vi "draw_3d_scene.vi"(4 "park plane z (px)":dbl=100.0, 5 "cells":dbl[][](array[numeric]), 6 "manip 4":dbl[][](array[numeric]), 7 "manip 1":dbl[][](array[numeric]), 8 "error in":errorcluster, 9 "manip 3":dbl[][](array[numeric]), 10 "manip 2":dbl[][](array[numeric]), 11 "3d graph":refnum<k7>) -> (0 "error out":errorcluster, 3 "currentState out":T1(array[cluster]))   [LabVIEW 2015]
uses:
  <vilib>/Platform/NI_3dgraph.lvlib
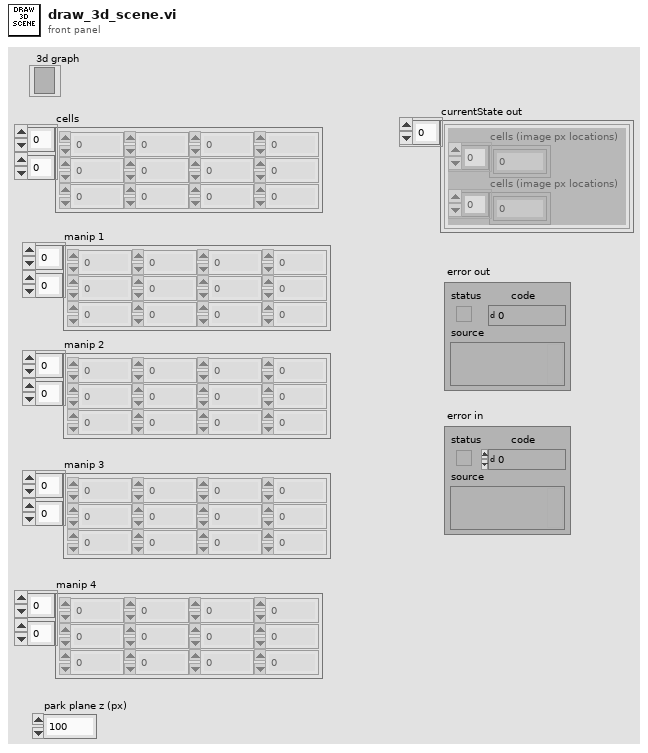
[diagram p1: front panel]
types:
  T1 = cluster{"cells (image px locations)":dbl[], "cells (image px locations)":dbl[]}[]
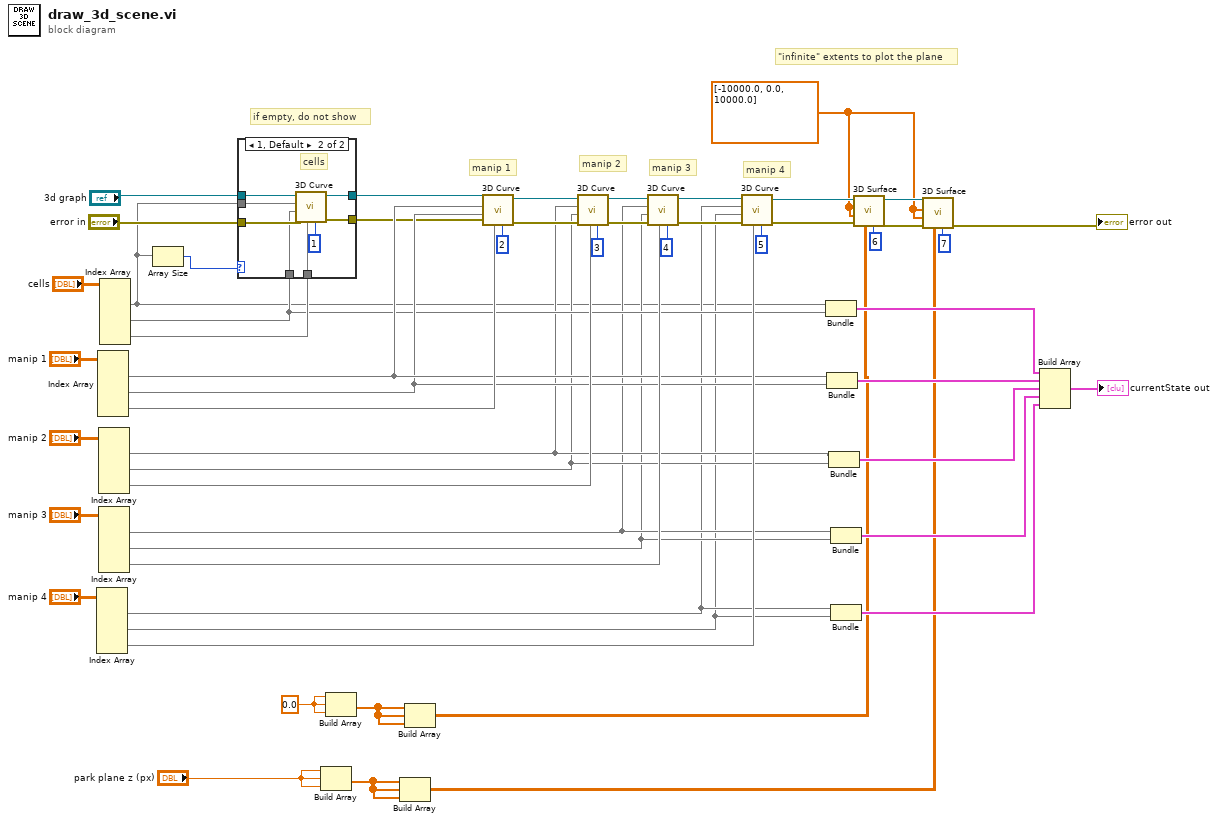
[diagram p0: block diagram]
diagram:
  w13 = 0.0 ("element")
  w6 = dbl[] [-10000.0, 0.0, 10000.0] ("x vector")
  # "if empty, do not show"
  # "\"infinite\" extents to plot the plane"
  # "manip 4"
  # "manip 3"
  # "manip 2"
  # "manip 1"
  n1 = Index Array(array="manip 4") -> (element #1=w21:dbl[], element #2=w20:dbl[], element #3=w41:dbl[])  [unwired: 6 in]
  n2 = Index Array(array="manip 1") -> (element #1=w36:dbl[], element #2=w35:dbl[], element #3=w47:dbl[])  [unwired: 6 in]
  n3 = Index Array(array="manip 2") -> (element #1=w26:dbl[], element #2=w25:dbl[], element #3=w43:dbl[])  [unwired: 6 in]
  n4 = Index Array(array="manip 3") -> (element #1=w23:dbl[], element #2=w22:dbl[], element #3=w42:dbl[])  [unwired: 6 in]
  n5 = Index Array(array="cells") -> (element #1=w1:dbl[], element #2=w28:dbl[], element #3=w29:dbl[])  [unwired: 6 in]
  n6 = Array Size(array=w1) -> (size(s)=w3:i32)
  n7 = case shown="1, Default" w3 {
    tunnel: "3d graph" -> [w57 w65]
    tunnel: "error in" -> [w56 w64]
    tunnel: [w56 w63] -> w31
    tunnel: [w57 w61] -> w30
    tunnel: w29 -> [_ w60]
    tunnel: w1 -> [_ w59]
    tunnel: w28 -> [_ w58]
    frame 0 {
    }
    frame 1, Default {
      # "cells"
      n8 = call <vilib>:"3D Curve.vi"("plot number (1)"=1, "z vector"=w60, "error in (no error)"=w64, "y vector"=w58, "x vector"=w59, "3D graph"=w65) -> ("error out"=w63:errorcluster, "3D graph out"=w61:refnum<k7>)  [unwired: 4 in]
    }
  }
  n9 = Build Array("park plane z (px)", "park plane z (px)", "park plane z (px)") -> (w9:dbl[])
  n10 = Build Array(w13, w13, w13) -> (w15:dbl[])
  n11 = Build Array(w9, w9, w9) -> (w7:dbl[][])
  n12 = Build Array(w15, w15, w15) -> (w14:dbl[][])
  n13 = call <vilib>:"3D Curve.vi"("plot number (1)"=2, "z vector"=w47, "error in (no error)"=w31, "y vector"=w35, "x vector"=w36, "3D graph"=w30) -> ("error out"=w49:errorcluster, "3D graph out"=w55:refnum<k7>)  [unwired: 4 in]
  n14 = call <vilib>:"3D Curve.vi"("plot number (1)"=3, "z vector"=w43, "error in (no error)"=w49, "y vector"=w25, "x vector"=w26, "3D graph"=w55) -> ("error out"=w39:errorcluster, "3D graph out"=w50:refnum<k7>)  [unwired: 4 in]
  n15 = call <vilib>:"3D Curve.vi"("plot number (1)"=4, "z vector"=w42, "error in (no error)"=w39, "y vector"=w22, "x vector"=w23, "3D graph"=w50) -> ("error out"=w38:errorcluster, "3D graph out"=w40:refnum<k7>)  [unwired: 4 in]
  n16 = call <vilib>:"3D Curve.vi"("plot number (1)"=5, "z vector"=w41, "error in (no error)"=w38, "y vector"=w20, "x vector"=w21, "3D graph"=w40) -> ("error out"=w16:errorcluster, "3D graph out"=w17:refnum<k7>)  [unwired: 4 in]
  n17 = Bundle("cells"=w1, "cells"=w28) -> (w27:cluster{"cells":dbl[], "cells":dbl[]})  [unwired: 1 in]
  n18 = Bundle("manip 1"=w36, "manip 1"=w35) -> (w34:cluster{"manip 1":dbl[], "manip 1":dbl[]})  [unwired: 1 in]
  n19 = Bundle("manip 2"=w26, "manip 2"=w25) -> (w24:cluster{"manip 2":dbl[], "manip 2":dbl[]})  [unwired: 1 in]
  n20 = Bundle("manip 3"=w23, "manip 3"=w22) -> (w19:cluster{"manip 3":dbl[], "manip 3":dbl[]})  [unwired: 1 in]
  n21 = Bundle("manip 4"=w21, "manip 4"=w20) -> (w18:cluster{"manip 4":dbl[], "manip 4":dbl[]})  [unwired: 1 in]
  n22 = call <vilib>:"3D Surface.vi"("plot number (1)"=6, "z matrix"=w14, "error in (no error)"=w16, "y vector"=w6, "x vector"=w6, "3D graph"=w17) -> ("error out"=w12:errorcluster, "3D graph out"=w10:refnum<k7>)  [unwired: 4 in]
  n23 = call <vilib>:"3D Surface.vi"("plot number (1)"=7, "z matrix"=w7, "error in (no error)"=w12, "y vector"=w6, "x vector"=w6, "3D graph"=w10) -> ("error out"=→"error out":errorcluster)  [unwired: 4 in, 1 out]
  n24 = Build Array(w27, w34, w24, w19, w18) -> (→"currentState out":cluster{"manip 4":dbl[], "manip 4":dbl[]}[])
